vi "Init WebView2 Core.vi"(8 "error in (no error)":errorcluster, 10 "Display State In":T1, 11 ".NET Refnum in":refnum<k24>) -> (0 "error out":errorcluster, 2 "Display State In 2":T1={"WebView2 Ref"=refnum, "event callback refnum"=refnum, "Events"={"Navigation Complete Event"=refnum, "Source Changed Event"=refnum, "Document Title Changed Event"=refnum, "Status Bar Text Changed"=refnum, "Web Message Received"=refnum, "Window Close Requested"=refnum}, "Paths"={"Webview2 Native"=path "C:/Users/kleins/Desktop/webview2/microsoft.web.webview2.1.0.1370.28/build/native", "Edge Application"=path "", "User Data"=path ""}}, 3 ".NET Refnum out":refnum<k24>)   [LabVIEW 2020, in "WebView2 Control.xctl"]
uses:
  WebView2 Control.xctl
  E:/Labview/LV 2020/Libs/LV-WebView2/microsoft.web.webview2/lib/net45/Microsoft.Web.WebView2.Core.dll
  microsoft.web.webview2/lib/net45/Microsoft.Web.WebView2.Core.dll
  State.ctl
  E:/Labview/LV 2020/Libs/LV-WebView2/microsoft.web.webview2/lib/net45/Microsoft.Web.WebView2.WinForms.dll
  microsoft.web.webview2/lib/net45/Microsoft.Web.WebView2.WinForms.dll
  Paths.ctl
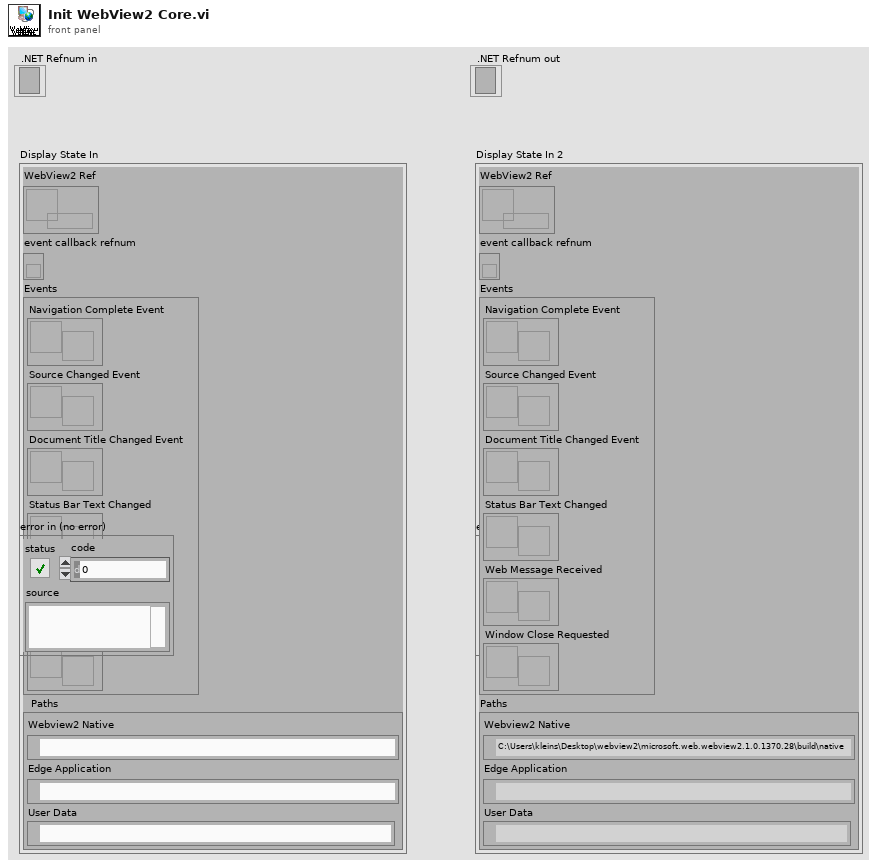
[diagram p1: front panel]
types:
  T1 = typedef "WebView2 Control.xctl/State.ctl" = cluster{"WebView2 Ref":refnum<data-value>, "event callback refnum":refnum<k27>, "Events":cluster{"Navigation Complete Event":refnum<user-event>, "Source Changed Event":refnum<user-event>, "Document Title Changed Event":refnum<user-event>, "Status Bar Text Changed":refnum<user-event>, "Web Message Received":refnum<user-event>, "Window Close Requested":refnum<user-event>}, "Paths":T2}
  T2 = typedef "WebView2 Control.xctl/Paths.ctl" = cluster{"Webview2 Native":path, "Edge Application":path, "User Data":path}
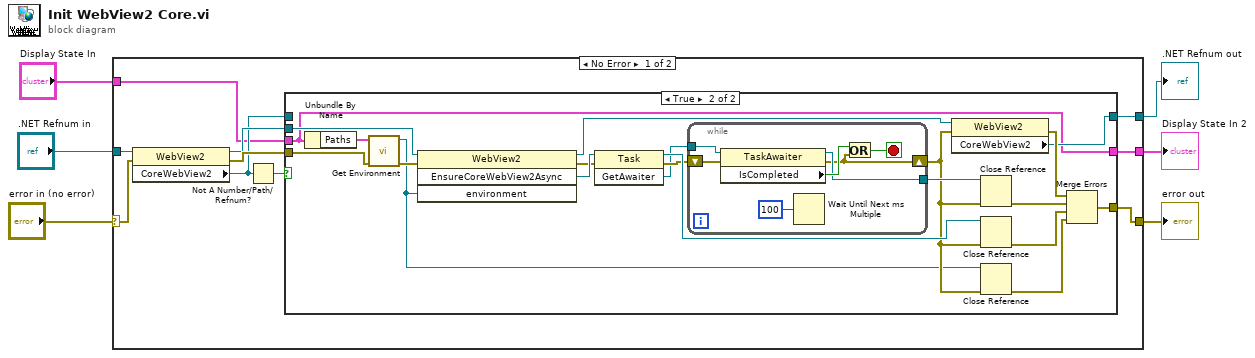
[diagram p0: block diagram]
diagram:
  n1 = case shown="No Error" "error in (no error)" {
    selector: "error in (no error)" -> [w9 w48]
    tunnel: [w16 _] -> w6
    tunnel: [w14 w48] -> w5
    tunnel: ".NET Refnum in" -> [w10 _]
    tunnel: [w8 w47] -> w2
    tunnel: "Display State In" -> [w7 w47]
    frame No Error {
      n2 = property class="WebView2"(reference=w10, error in=w9) -> (reference out=w13:refnum<k24>, error out=w15:errorcluster, "CoreWebView2"=w12:refnum<k24>)
      n3 = Not A Number/Path/Refnum?(number/path/refnum=w12) -> (NaN/Path/Refnum?=w11:bool)
      n4 = case shown="True" w11 {
        tunnel: [w19 w25] -> w16
        tunnel: w12 -> [w19 _]
        tunnel: w13 -> [_ w31]
        tunnel: w7 -> [w17 w24]
        tunnel: w15 -> [w18 w22]
        tunnel: [w18 w26] -> w14
        tunnel: [w17 w24] -> w8
        frame False {
        }
        frame True {
          n5 = Unbundle By Name(w24) -> ("Paths"=w23:T2)
          n6 = call "Get Environment.vi"("error in"=w22, "Paths"=w23) -> ("error out"=w21:errorcluster, "Environment out"=w20:refnum<k24>)  [unwired: 8 in]
          n7 = invoke class="WebView2" method="EnsureCoreWebView2Async"(reference=w31, error in=w21, "environment"=w20) -> (reference out=w38:refnum<k24>, error out=w36:errorcluster, "EnsureCoreWebView2Async"=w37:refnum<k24>)  [unwired: 1 in, 1 out]
          n8 = invoke class="Task" method="GetAwaiter"(reference=w37, error in=w36) -> (reference out=w35:refnum<k24>, error out=w30:errorcluster, "GetAwaiter"=w29:refnum<k24>)  [unwired: 1 in]
          n9 = while {
            tunnel: w29 -> [w45]
            shift-right: [w40] -> w27
            shift-left: w30 -> [w46]
            tunnel: [w42] -> w33
            stop <- w41 stop-if-true
            n10 = property class="TaskAwaiter"(reference=w45, error in=w46) -> (reference out=w42:refnum<k24>, error out=w40:errorcluster, "IsCompleted"=w43:bool)
            n11 = Wait Until Next ms Multiple(millisecond multiple=u32 100) -> ()  [unwired: 1 out]
            n12 = Or(x=w43, y=w40) -> (x .or. y?=w41:bool)
          }
          n13 = property class="WebView2"(reference=w38, error in=w27) -> (error out=w39:errorcluster, "CoreWebView2"=w25:refnum<k24>)  [unwired: 1 out]
          n14 = Close Reference(reference=w33, error in (no error)=w27) -> (error out=w32:errorcluster)
          n15 = Close Reference(reference=w35, error in (no error)=w27) -> (error out=w34:errorcluster)
          n16 = Close Reference(reference=w20, error in (no error)=w27) -> (error out=w28:errorcluster)
          n17 = Merge Errors(w39, w32, w34, w28) -> (w26:errorcluster)
        }
      }
    }
    frame Error {
    }
  }
  ".NET Refnum out" <- w6
  "error out" <- w5
  "Display State In 2" <- w2
